vi "Find Project Item.vi"(7 "Type":string, 8 "error in (no error)":errorcluster, 9 "Item Name":string, 10 "Target Name":string, 11 "Project Sync Tools in":refnum<class "Project Sync Tools.lvclass">) -> (0 "error out":errorcluster, 1 "Found ?":bool, 2 "ProjectItem out":refnum<vi>, 3 "Project Sync Tools out":refnum<class "Project Sync Tools.lvclass">)   [LabVIEW 2019, in "Project Sync Tools.lvclass"]
uses:
  Project Sync Tools.lvclass
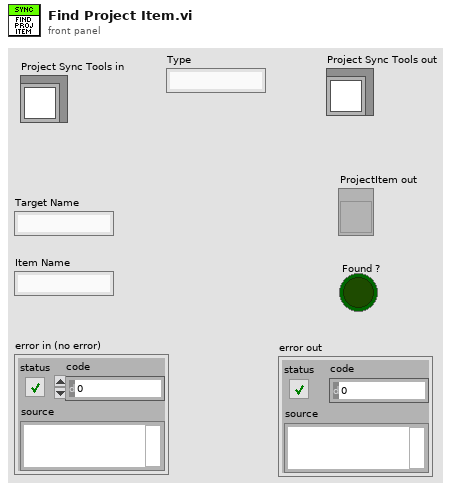
[diagram p1: front panel]
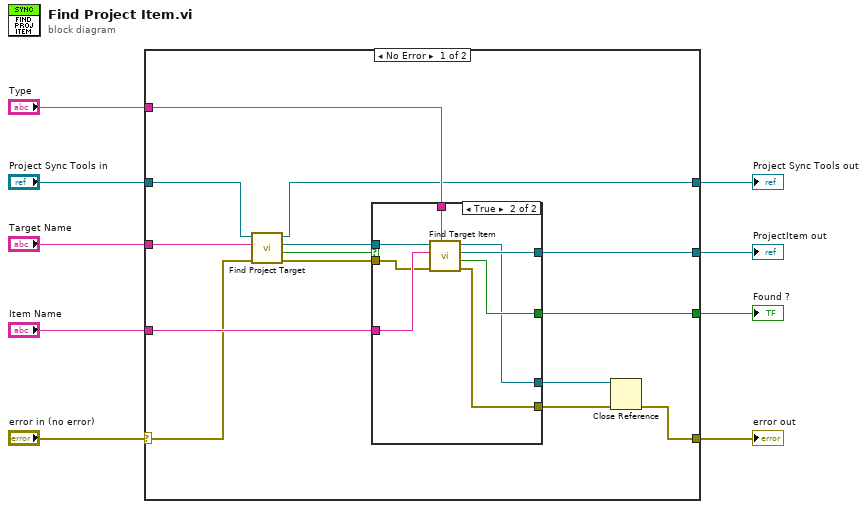
[diagram p0: block diagram]
diagram:
  n1 = case shown="No Error" "error in (no error)" {
    selector: "error in (no error)" -> [w17 w35]
    tunnel: [w23 _] -> w9
    tunnel: "Item Name" -> [w22 _]
    tunnel: "Target Name" -> [w20 _]
    tunnel: "Project Sync Tools in" -> [w11 w34]
    tunnel: [w10 w34] -> w5
    tunnel: [w14 w35] -> w3
    tunnel: [w16 _] -> w2
    tunnel: "Type" -> [w12 _]
    frame No Error {
      n2 = call "Find Project Target.vi"("error in (no error)"=w17, "Target Name"=w20, "Project Sync Tools in"=w11) -> ("error out"=w19:errorcluster, "Found ?"=w18:bool, "TargetItem out"=w21:refnum<vi>, "Project Sync Tools out"=w10:refnum<class "Project Sync Tools.lvclass">)  [unwired: 5 in]
      n3 = case shown="True" w18 {
        tunnel: [_ w33] -> w23
        tunnel: w22 -> [_ w32]
        tunnel: w21 -> [w24 w31]
        tunnel: w19 -> [w25 w27]
        tunnel: [w25 w30] -> w15
        tunnel: [_ w29] -> w16
        tunnel: [w24 w28] -> w13
        tunnel: w12 -> [_ w26]
        frame False {
        }
        frame True {
          n4 = call "Find Target Item.vi"("Type"=w26, "error in (no error)"=w27, "Target Item Name"=w32, "TargetItem in"=w31) -> ("error out"=w30:errorcluster, "Found ?"=w29:bool, "Item out"=w33:refnum<vi>, "TargetItem out"=w28:refnum<vi>)  [unwired: 4 in]
        }
      }
      n5 = Close Reference(reference=w13, error in (no error)=w15) -> (error out=w14:errorcluster)
    }
    frame Error {
    }
  }
  "ProjectItem out" <- w9
  "Project Sync Tools out" <- w5
  "error out" <- w3
  "Found ?" <- w2
